vi "Order Crossover.vi"(9 "Parent 2":T1, 10 "Parent 1":T1) -> (1 "Child 2":T1, 2 "Child 1":T1)   [LabVIEW 2013, in "GA.lvclass"]
uses:
  GA.lvclass
  Controls/Solution_GA.ctl
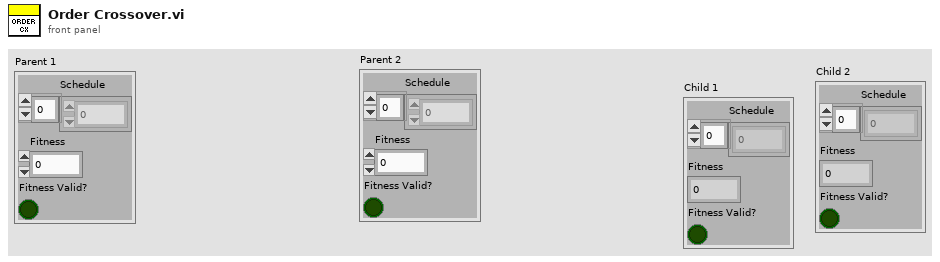
[diagram p1: front panel]
types:
  T1 = typedef "Solution_GA.ctl" = cluster{"Schedule":u16[], "Fitness":u16, "Fitness Valid?":bool}
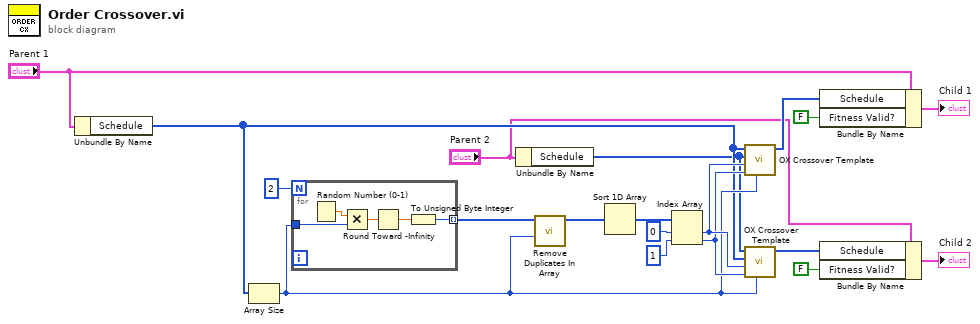
[diagram p0: block diagram]
diagram:
  n1 = Unbundle By Name("Parent 1") -> ("Schedule"=w5:u16[])
  n2 = Array Size(array=w5) -> (size(s)=w17:i32)
  n3 = for {
    N: 2 -> [_]
    tunnel: w17 -> [w23]
    tunnel: [w20] -> w11 mode=indexing
    n4 = Random Number (0-1)() -> (number: 0 to 1=w24:dbl)
    n5 = Multiply(x=w24, y=w23) -> (x*y=w22:dbl)
    n6 = Round Toward -Infinity(1:w22) -> (0:w21:dbl)
    n7 = To Unsigned Byte Integer(number=w21) -> (unsigned 8bit integer=w20:u8)
  }
  n8 = Unbundle By Name("Parent 2") -> ("Schedule"=w3:u16[])
  n9 = call "Remove Duplicates In Array.vi"("Max Index Bound"=w17, "Random Numbers Array"=w11) -> ("Random Numbers Array without Duplicates"=w10:i32[])  [unwired: 9 in]
  n10 = Sort 1D Array(array=w10) -> (sorted array=w9:i32[])
  n11 = Index Array(array=w9, index #1=0 ("index"), index #2=1 ("index")) -> (element #1=w19:i32, element #2=w18:i32)
  n12 = call "OX Crossover Template.vi"("Array Size"=w17, "Index 2"=w18, "Index 1"=w19, "Schedule 2"=w3, "Schedule 1"=w5) -> ("Child"=w15:u16[])  [unwired: 6 in]
  n13 = call "OX Crossover Template.vi"("Array Size"=w17, "Index 2"=w18, "Index 1"=w19, "Schedule 2"=w5, "Schedule 1"=w3) -> ("Child"=w14:u16[])  [unwired: 6 in]
  n14 = Bundle By Name(cluster="Parent 1", "Schedule"=w15, "Fitness Valid?"=FALSE) -> (→"Child 1":T1)
  n15 = Bundle By Name(cluster="Parent 2", "Schedule"=w14, "Fitness Valid?"=FALSE) -> (→"Child 2":T1)
